vi "RTD_get_4wR.vi"(7 "type":T1=enum."COMET Tx5xx (ethernet)" caption="Type", 8 "error in":errorcluster, 10 "timeout [ms]":i32=5000, 11 "VISA in":refnum<visa-resource-name>) -> (0 "error out":errorcluster, 2 "R value [Ohm]":dbl, 3 "VISA out":refnum<visa-resource-name>)   [LabVIEW 2020]
uses:
  thermo_types.ctl
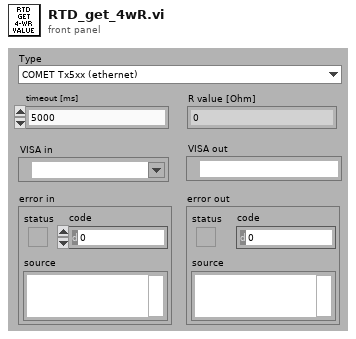
[diagram p1: front panel]
types:
  T1 = typedef "thermo_types.ctl" = enum16{"Disabled", "Simulated", "COMET Tx5xx (ethernet)", "Keithley 2002 (GPIB) + RTD", "Agilent 344xx (GPIB) + RTD"}
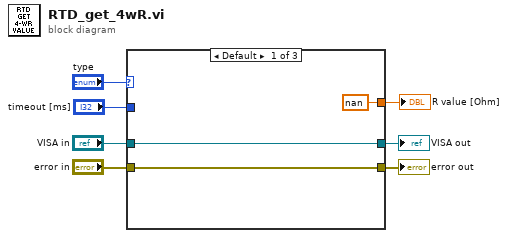
[diagram p0: block diagram]
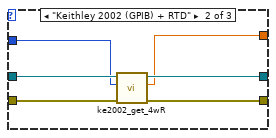
[diagram p2: hidden frame]
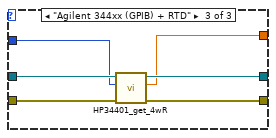
[diagram p3: hidden frame]
diagram:
  n1 = case shown="Default" "type" {
    tunnel: "error in" -> [w10 w16 w22]
    tunnel: [w10 w14 w20] -> w5
    tunnel: [w9 w13 w19] -> w4
    tunnel: "VISA in" -> [w9 w15 w21]
    tunnel: [nan ("Measurement") w12 w18] -> w2
    tunnel: "timeout [ms]" -> [_ w11 w17]
    frame Default {
    }
    frame "Keithley 2002 (GPIB) + RTD" {
      n2 = call "ke2002_get_4wR.vi"("error in"=w16, "timeout [ms]"=w11, "VISA in"=w15) -> ("error out"=w14:errorcluster, "R value [Ohm]"=w12:dbl, "VISA out"=w13:refnum<visa-resource-name>)  [unwired: 6 in]
    }
    frame "Agilent 344xx (GPIB) + RTD" {
      n3 = call "HP34401_get_4wR.vi"("error in"=w22, "timeout [ms]"=w17, "VISA in"=w21) -> ("error out"=w20:errorcluster, "Measurement"=w18:dbl, "VISA out"=w19:refnum<visa-resource-name>)  [unwired: 6 in]
    }
  }
  "error out" <- w5
  "VISA out" <- w4
  "R value [Ohm]" <- w2
